vi "BeamGage Callback with notification.vi"(4 "User Parameter":T1, 6 "Control Ref":refnum<k24>, 7 "Event Common Data":T2) -> ()   [LabVIEW 2019]
doc: "A .net callback VI that queries BeamGage for measurements results and frame data. The output is loaded into a notifier queue than can be read by an upper level VI as new results become available."
uses:
  C:/Program Files/Spiricon/BeamGage Professional/Spiricon.BeamGage.Automation.dll
  Spiricon.BeamGage.Automation.dll
  C:/Program Files/Spiricon/BeamGage Professional/Spiricon.Automation.dll
  Spiricon.Automation.dll
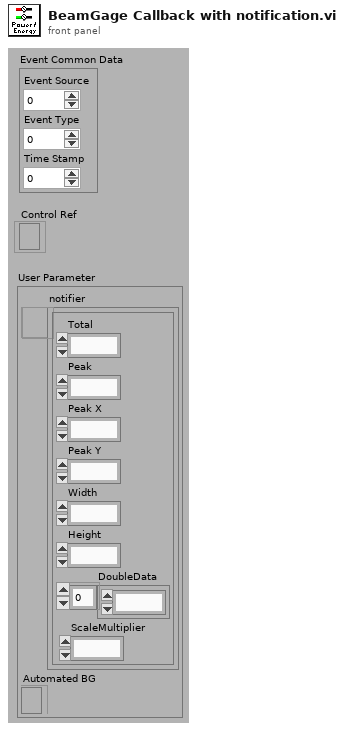
[diagram p1: front panel]
types:
  T1 = cluster{"notifier":refnum<notifier>, "Automated BG":refnum<k24>}
  T2 = cluster{"Event Source":i32, "Event Type":u32, "Time Stamp":u32}
  T3 = cluster{"Total":dbl, "Peak":dbl, "PeakLocationX":dbl, "PeakLocationY":dbl, "Width":dbl, "Height":dbl, "DoubleData":dbl[], "ScaleMultiplier":dbl}
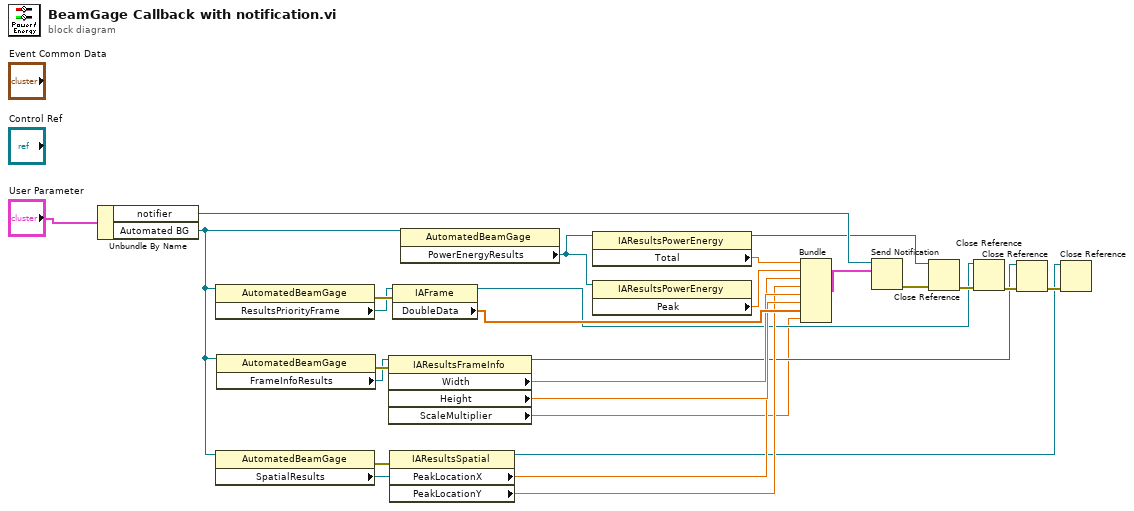
[diagram p0: block diagram]
diagram:
  n1 = Unbundle By Name("User Parameter") -> ("notifier"=w25:refnum<notifier>, "Automated BG"=w2:refnum<k24>)
  n2 = property class="AutomatedBeamGage"(reference=w2) -> (error out=w20:errorcluster, "ResultsPriorityFrame"=w8:refnum<k24>)  [unwired: 1 in, 1 out]
  n3 = property class="AutomatedBeamGage"(reference=w2) -> (error out=w15:errorcluster, "SpatialResults"=w6:refnum<k24>)  [unwired: 1 in, 1 out]
  n4 = property class="AutomatedBeamGage"(reference=w2) -> (error out=w18:errorcluster, "FrameInfoResults"=w7:refnum<k24>)  [unwired: 1 in, 1 out]
  n5 = property class="IAResultsFrameInfo"(reference=w7, error in=w18) -> (reference out=w5:refnum<k24>, "Width"=w17:dbl, "Height"=w16:dbl, "ScaleMultiplier"=w1:dbl)  [unwired: 1 out]
  n6 = property class="IAResultsSpatial"(reference=w6, error in=w15) -> (reference out=w4:refnum<k24>, "PeakLocationX"=w14:dbl, "PeakLocationY"=w13:dbl)  [unwired: 1 out]
  n7 = property class="IAFrame"(reference=w8, error in=w20) -> (reference out=w3:refnum<k24>, "DoubleData"=w19:dbl[])  [unwired: 1 out]
  n8 = property class="AutomatedBeamGage"(reference=w2) -> ("PowerEnergyResults"=w22:refnum<k24>)  [unwired: 1 in, 2 out]
  n9 = property class="IAResultsPowerEnergy"(reference=w22) -> (reference out=w21:refnum<k24>, "Total"=w24:dbl)  [unwired: 1 in, 1 out]
  n10 = property class="IAResultsPowerEnergy"(reference=w22) -> ("Peak"=w23:dbl)  [unwired: 1 in, 2 out]
  n11 = Bundle("Total"=w24, "Peak"=w23, "PeakLocationX"=w14, "PeakLocationY"=w13, "Width"=w17, "Height"=w16, "DoubleData"=w19, "ScaleMultiplier"=w1) -> (w12:T3)  [unwired: 1 in]
  n12 = Send Notification(notification=w12, notifier=w25) -> (error out=w27:errorcluster)  [unwired: 1 in, 1 out]
  n13 = Close Reference(reference=w21, error in (no error)=w27) -> (error out=w11:errorcluster)
  n14 = Close Reference(reference=w3, error in (no error)=w11) -> (error out=w10:errorcluster)
  n15 = Close Reference(reference=w5, error in (no error)=w10) -> (error out=w9:errorcluster)
  n16 = Close Reference(reference=w4, error in (no error)=w9) -> ()  [unwired: 1 out]
